vi "Base_get.vi"(8 "error in (no error)":errorcluster caption="错误输入（无错误）", 10 "buffer":string caption="缓冲区", 11 "url":string) -> (0 "error out":errorcluster caption="错误输出", 1 "body":string caption="体部", 2 "headers":string caption="头部")   [LabVIEW 2012, in "Http.lvclass"]
uses:
  Http.lvclass
  <vilib>/httpClient/POSTBuffer.vi
  <vilib>/httpClient/LabVIEWHTTPClient.lvlib
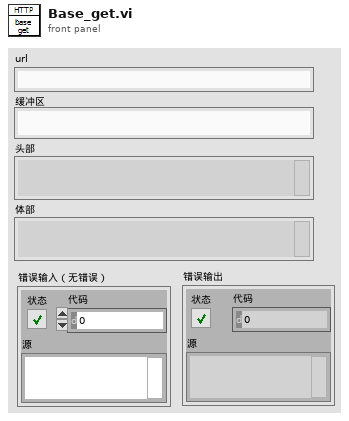
[diagram p1: front panel]
types:
  T1 = typedef "LabVIEWHTTPClient.lvlib/ClientHandle.ctl" = refnum<k1>
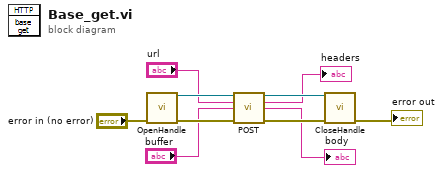
[diagram p0: block diagram]
diagram:
  n1 = call <vilib>:"OpenHandle.vi"("error in (no error)"="error in (no error)") -> ("client handle out"=w10:T1, "error out"=w9:errorcluster)  [unwired: 13 in]
  n2 = call-poly <vilib>:"POST.vi"("client handle"=w10, "url"="url", "buffer"="buffer", "error in (no error)"=w9) -> ("client handle out"=w8:T1, "headers"=→"headers":string, "body"=→"body":string, "error out"=w7:errorcluster)  [unwired: 8 in]
  n3 = call <vilib>:"CloseHandle.vi"("client handle"=w8, "error in (no error)"=w7) -> ("error out"=→"error out":errorcluster)  [unwired: 13 in]
